vi "Write CAN Spreadsheet.vi"(4 "transpose? (no:F)":bool, 5 "format (%s)":string="%s", 8 "error in":errorcluster, 9 "1D data":string[](array[string]), 10 "2D data":string[][](array[string]), 11 "file path":path) -> (0 "error out":errorcluster, 3 "new file path (Not A Path if cancelled)":path)   [LabVIEW 2010, in "CAN Log Transfer and Convert.lvlib"]
doc: "Converts a 2D or 1D array of strings, signed integers, or double-precision numbers to a text string and writes the string to a new byte stream file or appends the string to an existing file. Wire data to the <B>2D data</B> input or <B>1D data</B> input to determine the polymorphic instance to use or manually select the instance.\n\nUse this VI to transpose or separate data.\n\n<B>Note</B> To format with Microsoft Excel, use ActiveX with LabVIEW or the Report Generation Toolkit for Microsoft Office."
uses:
  CAN Log Transfer and Convert.lvlib
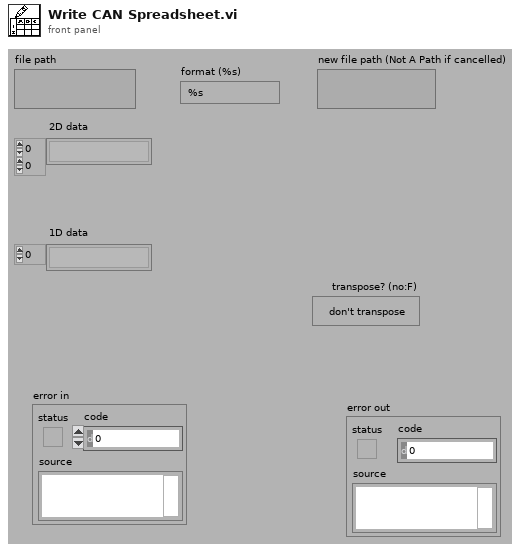
[diagram p1: front panel]
types:
  T1 = enum16{"open", "replace", "create", "open or create", "replace or create", "replace or create with confirmation"}
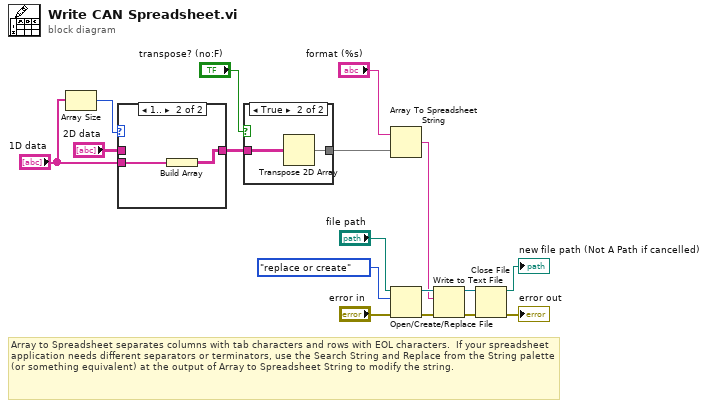
[diagram p0: block diagram]
diagram:
  # "Array to Spreadsheet separates columns with tab characters and rows with EOL characters.  If your spreadsheet application needs different separators or terminators, use the Search String and Replace from the String palette (or something equivalent) at the output of Array to Spreadsheet String to modify the string."
  n1 = Array Size(array="1D data") -> (size(s)=w17:i32)
  n2 = case shown="1.." w17 {
    tunnel: "1D data" -> [_ w20]
    tunnel: [w18 w19] -> w13
    tunnel: "2D data" -> [w18 _]
    frame ..0 {
      # "1D array is empty"
    }
    frame 1.. {
      n3 = Build Array(w20) -> (w19:string[][])
    }
  }
  n4 = case shown="True" "transpose? (no:F)" {
    tunnel: [w21 w23] -> w11
    tunnel: w13 -> [w21 w22]
    frame False {
    }
    frame True {
      n5 = Transpose 2D Array(2D array=w22) -> (transposed array=w23:string[][])
    }
  }
  n6 = Array To Spreadsheet String(array=w11, 3:"format (%s)") -> (spreadsheet string=w3:string)  [unwired: 1 in]
  n7 = Open/Create/Replace File(file path (use dialog)="file path", error in="error in", operation (0:open)=T1."replace or create") -> (refnum out=w5:refnum<file>, error out=w6:errorcluster)  [unwired: 3 in, 1 out]
  n8 = Write to Text File(file (use dialog)=w5, text=w3, error in=w6) -> (refnum out=w9:refnum<file>, error out=w8:errorcluster)  [unwired: 1 in, 1 out]
  n9 = Close File(refnum=w9, error in=w8) -> (path=→"new file path (Not A Path if cancelled)":path, error out=→"error out":errorcluster)
